vi "Simulate_Do_Adam_Channel.vi"(2 "Scan Period":dbl=6.0 format="%.2f", 3 "Previuos Scan Value":dbl=6.0 format="%.2f", 4 "Ch values":dbl[](array[numeric])=[101.0, 215.0, 308.0, 400.0, 531.0, 602.0, 701.0, 803.0, 901.0, 1000.0, 1103.0, 1203.0, 1301.0, 1401.0, 0.0, 0.0, 8.0, 2.5, 2.5, 2.5, 2.5, 2.5, 2.5, 2.5, 325.99887632296395, 19.39158422152035, 2.2449597721846404, 0.5799554886211512, 0.03449783578759482, 0.003993807452030343, 2.526317971, 0.0, -72.46272598652615, 0.0, 0.0, 1.17497766, 32.240363150627225, 210.0, 1020.0, 301.0, 2.5, 142.10424331613308, 0.0, 328.2438360951486, 0.5839492960731816, 1.7790106983270548, 1.5193370165745854, 0.0, 0.6839305191199052, 25.05543717569892, 2.5, 1003.0, 2.5, 1.0, 1.0, 2.438043804, 12.768040386036008, 12.706066679299887, 1.5529939411190576, 1.6417227074933711, 1.577996015069992, 1.5379619305483683, 392.62743714012475, 391.12318614802876, 390.2349588262341, 393.196709833076, 2.5, 2.5, 2.5, 2.5, 2.5, 2.5, 25.319705293675124, 25.259814181650874, 25.12704771497858, 25.012422365813457, 25.293841944534957, 0.025863349140166747, 25.273768518626966, 40.104614519787646, 40.24383199536746, 40.13478438003449, 40.497608336401, 40.44780827684571, 40.31870788173805, 40.44582031947223, 40.309581705207755, 40.2223555477384, 40.372225710241445, 40.38773761174557, 40.15855495963509, 40.16015237958758, 40.468233934989506, 40.457340299586214, 40.315290523891875, 40.497608336401, 0.0, 40.36899533293672, 40.25203586968345, 40.0257139604184, 40.025198234250645, 40.17651039138312, 40.44097626352102, 40.05545286253188, 40.14486114776275, 40.334417441523165, 40.077317352292724, 40.430256065061144, 40.37289703400107, 40.227796869630744, 40.12172580298229, 40.23422587595286, 25.08701365883341, 25.259660230254553, 25.442317262985082, 25.26875092710488, 25.451964000408545, 25.496320648305083, 25.312010214521397, 25.401932174919292, 25.125518841017104, 25.14993274344684, 25.103609136185852, 25.477205373935536, 25.2202562728105, 25.406950290948178, 25.402628413785724, 25.22925712912244, 25.47194565357341, 25.388304574129034, 25.499521135726706, 25.04618408026844, 25.10219309451716, 25.224647136795284, 25.41004935241934, 25.41949341015379, 25.020688369766525, 25.476278977582126, 21.0, 100.0, 12.725703709925437, 25.21271246180679, 1.0, 25.39016376984826, 10.52, 12.716372991953591, 25.05543717569892] format="%.2f", 5 "Value to Output":dbl format="%.2f", 6 "Ch Discription":T1={"Ch Name"="", "Type"="", "Function"=enum."Analogue Input", "Ch State"=enum."On", "Calibration type"=enum."Raw", "A"=0.0, "B"=0.0, "C"=0.0, "D"=0.0, "Comments"="", "Address"={"Main"=0, "Ch."=0, "Sub"=0, "Port Name"=""}, "String"="", "Duty"=65535} {"Duty" format="%.0b"; "D" format="%#_5g"; "C" format="%#_5g"; "B" format="%#_5g"; "A" format="%#_5g"}, 7 "Ch names":string[](array[string])) -> (0 "Scan comment":string, 1 "Calibrated units":dbl=6.0 format="%.2f")   [LabVIEW 2012]
uses:
  ADAM Client/Sub VIs/ADAM Controls/Ch_description_ADAM.ctl
  ADAM Client/Sub VIs/ADAM Controls/Module_type_ADAM.ctl
  ADAM Client/Sub VIs/ADAM Controls/Function_ADAM.ctl
  ADAM Client/Sub VIs/ADAM Controls/Channel_State.ctl
  ADAM Client/Sub VIs/ADAM Controls/Calib_type_ADAM.ctl
  ADAM Client/Sub VIs/ADAM Controls/Address.ctl
panel:
  in  "Case Constant\n(See Context Help)":bool=TRUE
  in  "Gill Error":bool
  in  "Inlet Measured temp":dbl=25.0 format="%.2f"
  in  "4018 Temp":dbl=25.0 format="%.2f"
  in  "Default Output":dbl=2.5 format="%.2f"
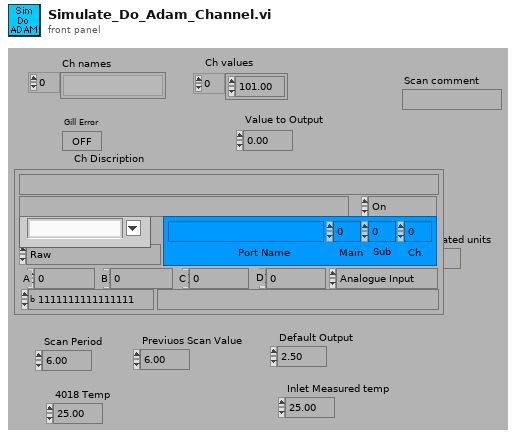
[diagram p1: front panel]
types:
  T1 = typedef "Ch_description_ADAM.ctl" = cluster{"Ch Name":string, "Type":T2, "Function":T3, "Ch State":T4, "Calibration type":T5, "A":dbl, "B":dbl, "C":dbl, "D":dbl, "Comments":string, "Address":T6, "String":string, "Duty":u16}
  T2 = typedef "Module_type_ADAM.ctl" = string
  T3 = typedef "Function_ADAM.ctl" = enum16{"Analogue Input", "Digital Input", "Event counter", "Event rate", "Analogue Output", "Digital Output", "Relay Output"}
  T4 = typedef "Channel_State.ctl" = enum16{"On", "Off", "Always On", "Always Off"}
  T5 = typedef "Calib_type_ADAM.ctl" = enum16{"Raw", "Bx + A", "Cx^2 + Bx + A", "Dx^3 + Cx^2 + Bx + A", "In Band", "Hi-Tec Q", "Hi-Tec M_dot", "Text"}
  T6 = typedef "Address.ctl" = cluster{"Main":i32, "Ch.":i32, "Sub":i32, "Port Name":string}
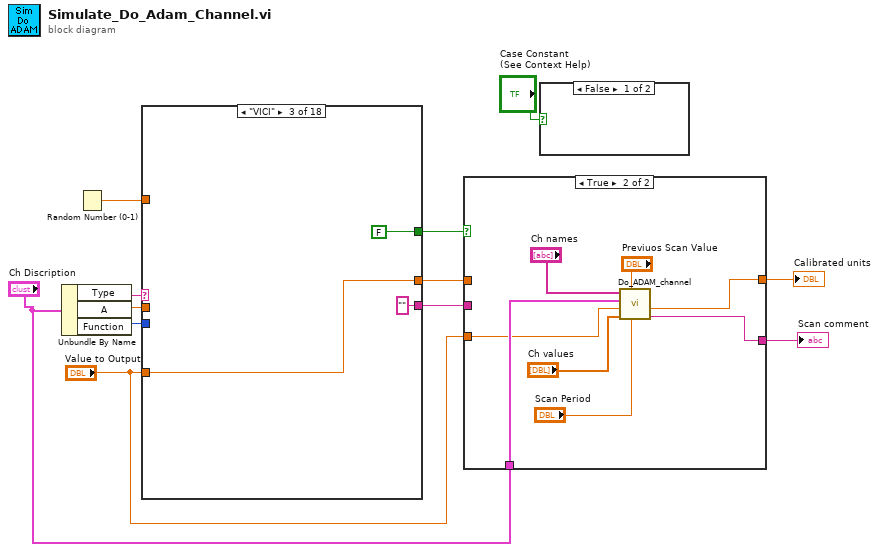
[diagram p0: block diagram]
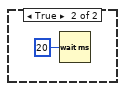
[diagram p2: hidden frame]
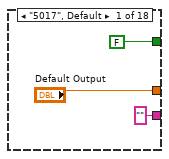
[diagram p4: hidden frame]
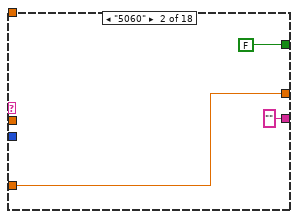
[diagram p5: hidden frame]
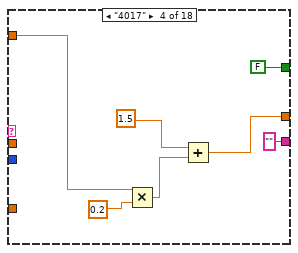
[diagram p6: hidden frame]
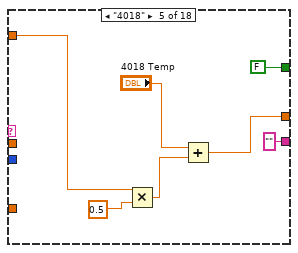
[diagram p7: hidden frame]
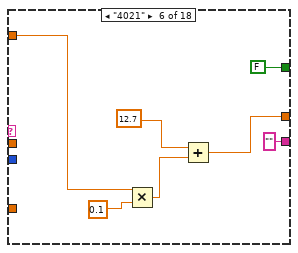
[diagram p8: hidden frame]
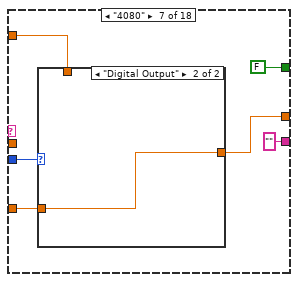
[diagram p9: hidden frame]
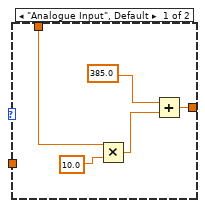
[diagram p10: hidden frame]
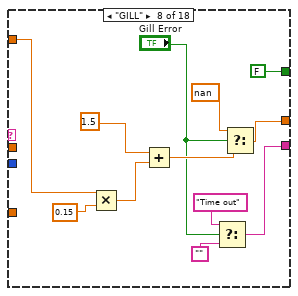
[diagram p11: hidden frame]
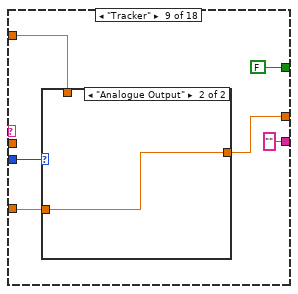
[diagram p12: hidden frame]
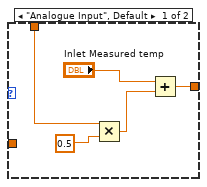
[diagram p13: hidden frame]
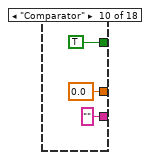
[diagram p14: hidden frame]
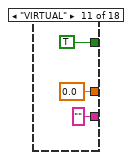
[diagram p15: hidden frame]
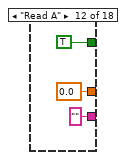
[diagram p16: hidden frame]
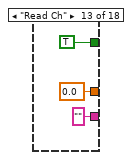
[diagram p17: hidden frame]
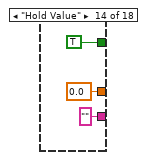
[diagram p18: hidden frame]
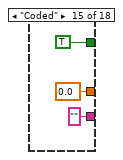
[diagram p19: hidden frame]
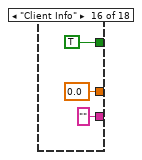
[diagram p20: hidden frame]
diagram:
  n1 = Unbundle By Name("Ch Discription") -> ("Type"=w12:T2, "A"=w5:dbl, "Function"=w3:T3)
  n2 = Random Number (0-1)() -> (number: 0 to 1=w7:dbl)
  n3 = case shown="\"VICI\"" w12 {
    tunnel: [FALSE FALSE FALSE FALSE FALSE FALSE FALSE FALSE FALSE TRUE TRUE TRUE TRUE TRUE TRUE TRUE FALSE TRUE] -> w8
    tunnel: w7 -> [_ _ _ w26 w33 w40 w47 w64 w71 _ _ _ _ _ _ _ _ _]
    tunnel: ["Default Output" w17 w20 w23 w31 w37 w46 w59 w70 0.0 0.0 0.0 0.0 0.0 0.0 0.0 1003.0 0.0] -> w6
    tunnel: w5 -> [_ _ _ _ _ _ _ _ _ _ _ _ _ _ _ _ _ _]
    tunnel: w3 -> [_ _ _ _ _ _ w45 _ w69 _ _ _ _ _ _ _ _ _]
    tunnel: "Value to Output" -> [_ w17 w20 _ _ _ w44 _ w68 _ _ _ _ _ _ _ _ _]
    tunnel: ["" ("Scan comment") "" ("Scan comment") "" ("Scan comment") "" ("Scan comment") "" ("Scan comment") "" ("Scan comment") "" ("Scan comment") w55 "" ("Scan comment") "" ("Scan comment") "" ("Scan comment") "" ("Scan comment") "" ("Scan comment") "" ("Scan comment") "" ("Scan comment") "" ("Scan comment") "" ("Scan comment") "" ("Scan comment")] -> w1
    frame "5017", Default {
    }
    frame "5060" {
    }
    frame "VICI" {
    }
    frame "4017" {
      n4 = Multiply(x=w26, y=0.2) -> (x*y=w25:dbl)
      n5 = Add(x=1.5, y=w25) -> (x+y=w23:dbl)
    }
    frame "4018" {
      n6 = Multiply(x=w33, y=0.5) -> (x*y=w32:dbl)
      n7 = Add(x="4018 Temp", y=w32) -> (x+y=w31:dbl)
    }
    frame "4021" {
      n8 = Multiply(x=w40, y=0.1) -> (x*y=w39:dbl)
      n9 = Add(x=12.7, y=w39) -> (x+y=w37:dbl)
    }
    frame "4080" {
      n10 = case shown="\"Digital Output\"" w45 {
        tunnel: w47 -> [w52 _]
        tunnel: [w49 w54] -> w46
        tunnel: w44 -> [_ w54]
        frame "Analogue Input", Default {
          n11 = Multiply(x=w52, y=10.0) -> (x*y=w51:dbl)
          n12 = Add(x=385.0, y=w51) -> (x+y=w49:dbl)
        }
        frame "Digital Output" {
        }
      }
    }
    frame "GILL" {
      n13 = Multiply(x=w64, y=0.15) -> (x*y=w63:dbl)
      n14 = Add(x=1.5, y=w63) -> (x+y=w61:dbl)
      n15 = Select(t="Time out" ("Scan comment"), s="Gill Error", f="") -> (s? t:f=w55:string)
      n16 = Select(t=nan, s="Gill Error", f=w61) -> (s? t:f=w59:dbl)
    }
    frame "Tracker" {
      n17 = case shown="\"Analogue Output\"" w69 {
        tunnel: w71 -> [w76 _]
        tunnel: [w74 w78] -> w70
        tunnel: w68 -> [_ w78]
        frame "Analogue Input", Default {
          n18 = Multiply(x=w76, y=0.5) -> (x*y=w75:dbl)
          n19 = Add(x="Inlet Measured temp", y=w75) -> (x+y=w74:dbl)
        }
        frame "Analogue Output" {
        }
      }
    }
    frame "Comparator" {
    }
    frame "VIRTUAL" {
    }
    frame "Read A" {
    }
    frame "Read Ch" {
    }
    frame "Hold Value" {
    }
    frame "Coded" {
    }
    frame "Client Info" {
    }
    frame "Web Client" {
    }
    frame "Test" {
    }
  }
  n20 = case shown="True" w8 {
    tunnel: "Ch Discription" -> [_ w114]
    tunnel: [w107 w110] -> w10
    tunnel: [w106 w109] -> w9
    tunnel: w6 -> [w107 _]
    tunnel: "Value to Output" -> [_ w108]
    tunnel: w1 -> [w106 _]
    frame False {
    }
    frame True {
      n21 = call "Do_ADAM_channel.vi"("Scan Period"="Scan Period", "Previous Scan Value"="Previuos Scan Value", "Present scan array"="Ch values", "Value to Output"=w108, "Ch Description"=w114, "Ch names"="Ch names") -> ("Scan comment"=w109:string, "Output"=w110:dbl)  [unwired: 2 out]
    }
  }
  "Calibrated units" <- w10
  "Scan comment" <- w9
  n22 = case shown="False" "Case Constant\n(See Context Help)" {
    frame False {
    }
    frame True {
      n23 = Wait (ms)(milliseconds to wait=u32 20) -> ()  [unwired: 1 out]
    }
  }
